vi "filter.vi"(10 "Array":dbl[][](array[numeric]), 11 "ori":T1) -> (3 "image data":T1)   [LabVIEW 2023]
doc: "Filters image. Input image and mask."
uses:
  <vilib>/picture/picture.llb/imagedata.ctl
  <vilib>/Analysis/2dsp.llb/2D Convolution (DBL).vi
  <vilib>/Analysis/NI_AALPro.lvlib
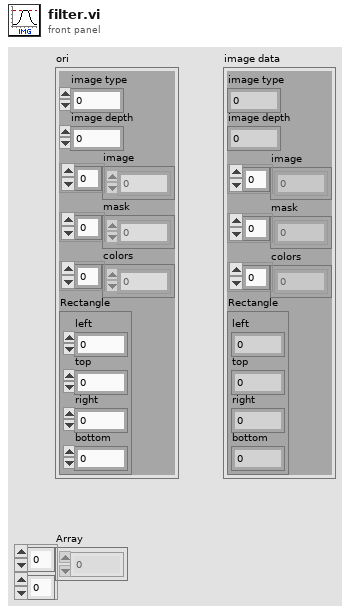
[diagram p1: front panel]
types:
  T1 = typedef "imagedata.ctl" = cluster{"image type":i32, "image depth":i32, "image":u8[], "mask":u8[], "colors":u32[], "Rectangle":cluster{"left":i16, "top":i16, "right":i16, "bottom":i16}}
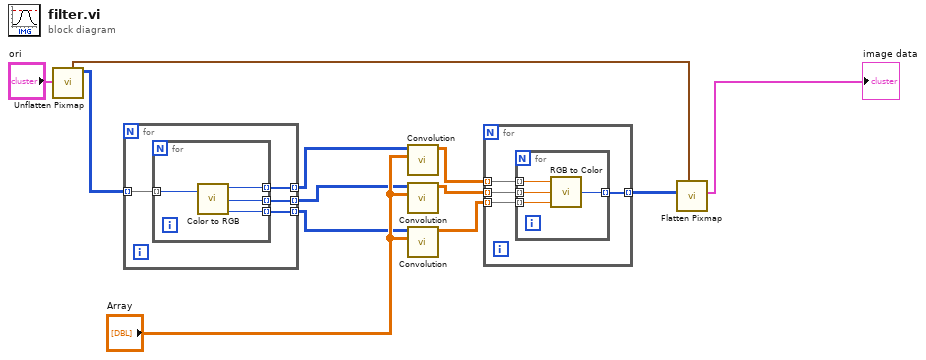
[diagram p0: block diagram]
diagram:
  n1 = call <vilib>:"Unflatten Pixmap.vi"("image data"="ori") -> ("24-bit pixmap"=w3:u32[][], "top left"=w1:cluster{"x":i16, "y":i16})  [unwired: 4 in, 5 out]
  n2 = for {
    tunnel: w3 -> [w16] mode=indexing
    tunnel: [w15] -> w4 mode=indexing
    tunnel: [w14] -> w5 mode=indexing
    tunnel: [w13] -> w6 mode=indexing
    n3 = for {
      tunnel: w16 -> [w20] mode=indexing
      tunnel: [w19] -> w15 mode=indexing
      tunnel: [w18] -> w14 mode=indexing
      tunnel: [w17] -> w13 mode=indexing
      n4 = call <vilib>:"Color to RGB.vi"("Color"=w20) -> ("R"=w19:u8, "G"=w18:u8, "B"=w17:u8)  [unwired: 1 out]
    }
  }
  n5 = call-poly <vilib>:"Convolution.vi"("Y"="Array", "X"=w4) -> ("X * Y"=w7:dbl[][])  [unwired: 8 in, 1 out]
  n6 = call-poly <vilib>:"Convolution.vi"("Y"="Array", "X"=w5) -> ("X * Y"=w8:dbl[][])  [unwired: 8 in, 1 out]
  n7 = call-poly <vilib>:"Convolution.vi"("Y"="Array", "X"=w6) -> ("X * Y"=w9:dbl[][])  [unwired: 8 in, 1 out]
  n8 = for {
    tunnel: w7 -> [w24] mode=indexing
    tunnel: w8 -> [w23] mode=indexing
    tunnel: w9 -> [w22] mode=indexing
    tunnel: [w21] -> w12 mode=indexing
    n9 = for {
      tunnel: w24 -> [w28] mode=indexing
      tunnel: w23 -> [w27] mode=indexing
      tunnel: w22 -> [w26] mode=indexing
      tunnel: [w25] -> w21 mode=indexing
      n10 = call <vilib>:"RGB to Color.vi"("B"=w26, "G"=w27, "R"=w28) -> ("Color"=w25:u32)
    }
  }
  n11 = call <vilib>:"Flatten Pixmap.vi"("top left"=w1, "24-bit pixmap"=w12) -> ("image data"=→"image data":T1)  [unwired: 9 in]
